vi "Module Identities.vi"(8 "error in (no error)":errorcluster, 11 "Role Manager in":refnum<class "Role Manager.lvclass">) -> (0 "error out":errorcluster, 2 "Identities":refnum<class "Identity.lvclass">[](array[class]), 3 "Role Manager out":refnum<class "Role Manager.lvclass">)   [LabVIEW 2020, in "Volatus.lvlib" / "Role Manager.lvclass"]
uses:
  Role Manager.lvclass
  Identity/Identity.lvclass
  Role Manager.lvclass/Role Manager.ctl
  Role Manager Identity/Role Manager Identity.lvclass
  C:/dev/lv20CE/relink/lv-volatus/Volatus/Role Manager Identity/Role Manager Identity.lvclass
  C:/dev/lv20CE/relink/lv-volatus/Volatus/Identity/Identity.lvclass
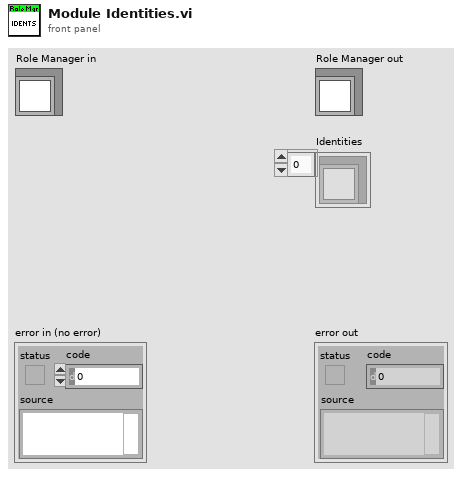
[diagram p1: front panel]
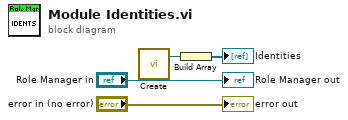
[diagram p0: block diagram]
diagram:
  n1 = call "Create.vi"() -> ("Role Manager Identity out"=w2:refnum<class "Role Manager Identity.lvclass">)  [unwired: 7 in]
  n2 = Build Array(w2) -> (→"Identities":refnum<class "Role Manager Identity.lvclass">[])
  "error out" <- "error in (no error)"
  "Role Manager out" <- "Role Manager in"
